vi "test Modify Alias and Endpoint.vi"(8 "error in (no error)":errorcluster, 11 "TestCase in":refnum<class "Routing and Faulting Scripting Unit Tests.lvclass">) -> (0 "error out":errorcluster, 3 "TestCase out":refnum<class "Routing and Faulting Scripting Unit Tests.lvclass">)   [LabVIEW 2017, in "Routing and Faulting Scripting Unit Tests.lvclass"]
uses:
  Routing and Faulting Scripting Unit Tests.lvclass
  Routing and Faulting Scripting Unit Tests.lvclass/Routing and Faulting Scripting Unit Tests.ctl
  <vilib>/addons/_JKI Toolkits/VI Tester/TestCase.llb/TestCase.lvclass
  Routing and Faulting Scripting.lvlib
  C:/Program Files (x86)/National Instruments/LabVIEW 2017/vi.lib/addons/_JKI Toolkits/VI Tester/TestCase.llb/TestCase.lvclass
panel:
  in  "Save?":bool
  out "Output Filename":string
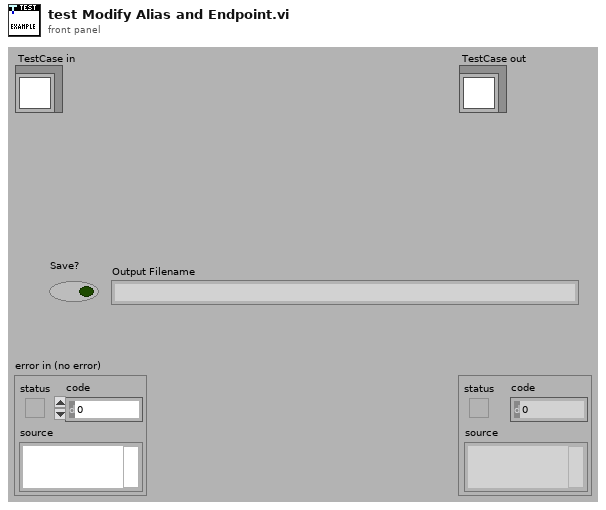
[diagram p1: front panel]
types:
  T1 = typedef "Custom Device API.lvlib/Custom Device Item Ref.ctl" = u64
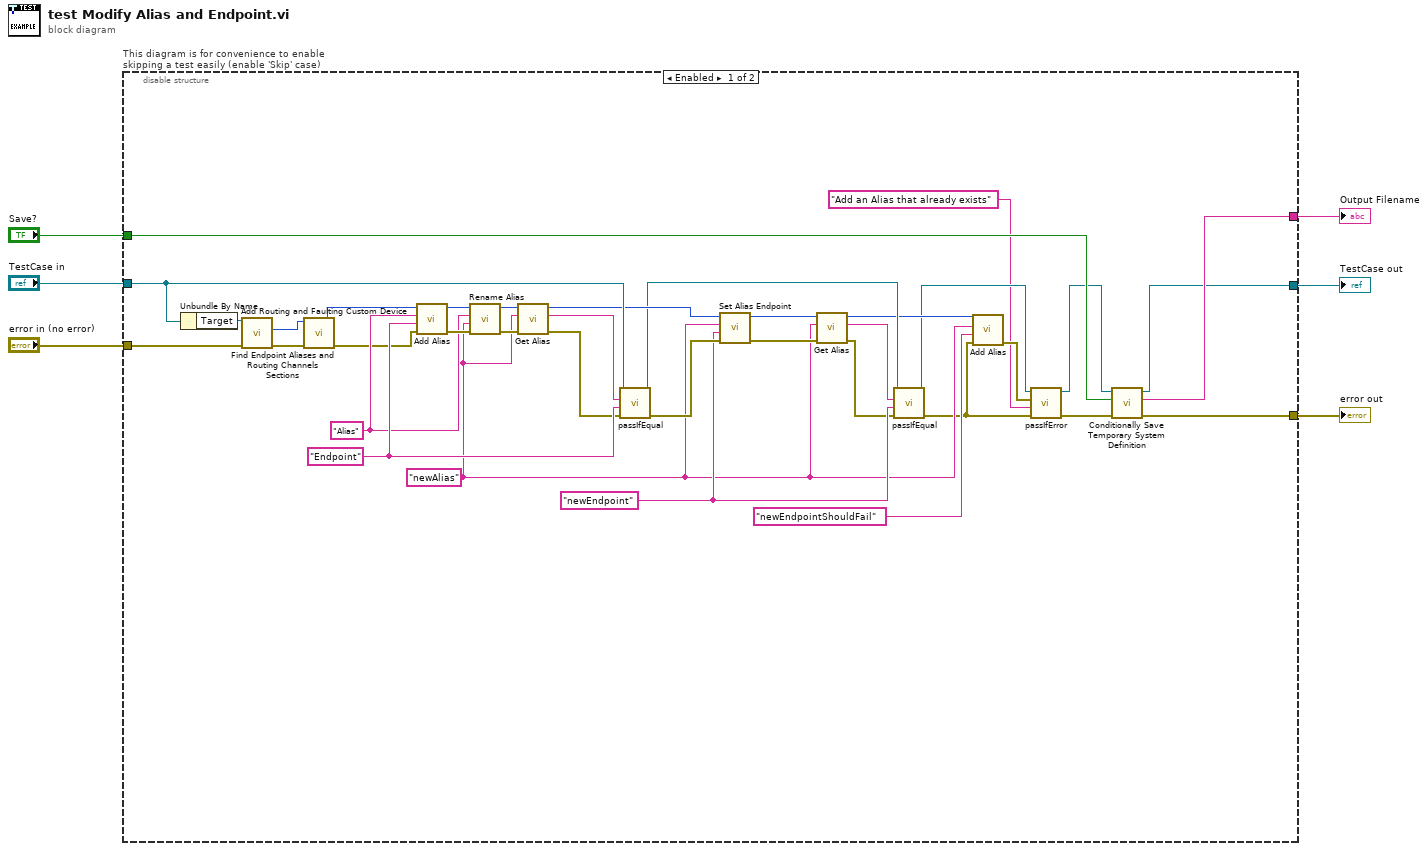
[diagram p0: block diagram]
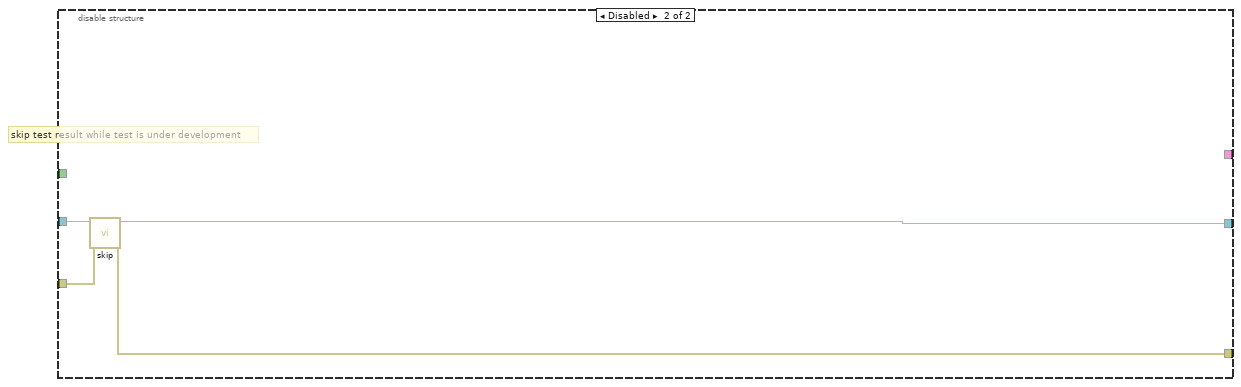
[diagram p2: hidden frame]
diagram:
  n1 = disable-structure "This diagram is for convenience to enable skipping a test easily (enable 'Skip' case)" shown="Enabled" {
    disable-tunnel: "TestCase in" -> [w37 w46]
    disable-tunnel: [w40 w44] -> w3
    disable-tunnel: [w41 w45] -> w5
    disable-tunnel: "error in (no error)" -> [w38 w43]
    disable-tunnel: [w42 _] -> w2
    disable-tunnel: "Save?" -> [w19 _]
    frame Enabled {
      w21 = "newEndpoint" ("Pin")
      w14 = "newAlias" ("Alias")
      w34 = "Endpoint" ("Pin")
      w28 = "Alias" ("Alias")
      n2 = Unbundle By Name(w37) -> ("Target"=w39:refnum<k24>)
      n3 = call "Add Routing and Faulting Custom Device.vi"("error in (no error)"=w38, "Target in"=w39) -> ("error out"=w36:errorcluster, "Routing and Faulting Custom Device Ref"=w17:T1)  [unwired: 7 in, 1 out]
      n4 = call "Find Endpoint Aliases and Routing Channels Sections.vi"("error in (no error)"=w36, "Routing and Faulting Custom Device Ref in"=w17) -> ("error out"=w18:errorcluster, "Endpoint Aliases Ref"=w16:T1)  [unwired: 6 in, 2 out]
      n5 = call "Add Alias.vi"("error in (no error)"=w18, "Endpoint"=w34, "Alias"=w28, "Endpoint Aliases Ref in"=w16) -> ("error out"=w30:errorcluster, "Endpoint Aliases Ref out"=w32:T1)  [unwired: 6 in]
      n6 = call "Rename Alias.vi"("error in (no error)"=w30, "New Alias Name"=w14, "Alias"=w28, "Endpoint Aliases Ref in"=w32) -> ("error out"=w29:errorcluster, "Endpoint Aliases Ref out"=w31:T1)  [unwired: 6 in]
      n7 = call "Get Alias.vi"("error in (no error)"=w29, "Alias"=w14, "Endpoint Aliases Ref in"=w31) -> ("error out"=w33:errorcluster, "Endpoint"=w35:string, "Endpoint Aliases Ref out"=w27:T1)  [unwired: 6 in]
      n8 = call-dynamic "passIfEqual.vi"("error in (no error)"=w33, "y"=w34, "x"=w35, "TestCase in"=w37) -> ("error out"=w26:errorcluster, "TestCase out"=w23:refnum<class "Routing and Faulting Scripting Unit Tests.lvclass">)  [unwired: 6 in]
      n9 = call "Set Alias Endpoint.vi"("error in (no error)"=w26, "New Endpoint"=w21, "Alias"=w14, "Endpoint Aliases Ref in"=w27) -> ("error out"=w24:errorcluster, "Endpoint Aliases Ref out"=w25:T1)  [unwired: 6 in]
      n10 = call "Get Alias.vi"("error in (no error)"=w24, "Alias"=w14, "Endpoint Aliases Ref in"=w25) -> ("error out"=w20:errorcluster, "Endpoint"=w22:string, "Endpoint Aliases Ref out"=w15:T1)  [unwired: 6 in]
      n11 = call-dynamic "passIfEqual.vi"("error in (no error)"=w20, "y"=w21, "x"=w22, "TestCase in"=w23) -> ("error out"=w11:errorcluster, "TestCase out"=w9:refnum<class "Routing and Faulting Scripting Unit Tests.lvclass">)  [unwired: 6 in]
      n12 = call "Add Alias.vi"("error in (no error)"=w11, "Endpoint"="newEndpointShouldFail" ("Pin"), "Alias"=w14, "Endpoint Aliases Ref in"=w15) -> ("error out"=w13:errorcluster)  [unwired: 6 in, 1 out]
      n13 = call-dynamic "passIfError.vi"("error in (no error)"=w11, "task (\"\")"="Add an Alias that already exists" ("task (\"\")"), "error"=w13, "TestCase in"=w9) -> ("error out"=w10:errorcluster, "TestCase out"=w8:refnum<class "Routing and Faulting Scripting Unit Tests.lvclass">)  [unwired: 6 in]
      n14 = call "Conditionally Save Temporary System Definition.vi"("error in (no error)"=w10, "Save?"=w19, "Test Case"=w8) -> ("error out"=w41:errorcluster, "filename"=w42:string, "Test Case"=w40:refnum<class "Routing and Faulting Scripting Unit Tests.lvclass">)  [unwired: 6 in]
    }
    frame Disabled {
      # "skip test result while test is under development"
      n15 = call <vilib>:"skip.vi"("error in (no error)"=w43, "TestCase in"=w46) -> ("error out"=w45:errorcluster, "TestCase out"=w44:refnum<class "Routing and Faulting Scripting Unit Tests.lvclass">)  [unwired: 8 in]
    }
  }
  "error out" <- w5
  "TestCase out" <- w3
  "Output Filename" <- w2
